vi "Main_old2.vi"() -> ()   [LabVIEW 2021]
uses:
  Enums/BatteryHealth_Enum.ctl
  Enums/Battery_Types.ctl
  Enums/States_Enum.ctl
  <vilib>/Utility/file.llb/Read Delimited Spreadsheet (DBL).vi
panel:
  out "counter":u8
  out "measurements done":u8
  out "Program State":T1
  in  "Battery Type":T2
  out "Quick Battery Health":T3
  out "error output":errorcluster
  in  "Stop Measurement":bool
  out "Battery Percentage":dbl caption="%" format="%#_2g%%"
  out "Internal Resistance":dbl format="%#_gohm"
  in  "Start Measurement":bool
  out "Battery Percentage Meter":dbl(knob)=21.586596923816817 caption="Meter" scale=0.0..100.0 scale format="%#_3g"
  out "read config":dbl[](array[numeric])
  out "read ascii file error":errorcluster
  in  "Terminate Run":bool
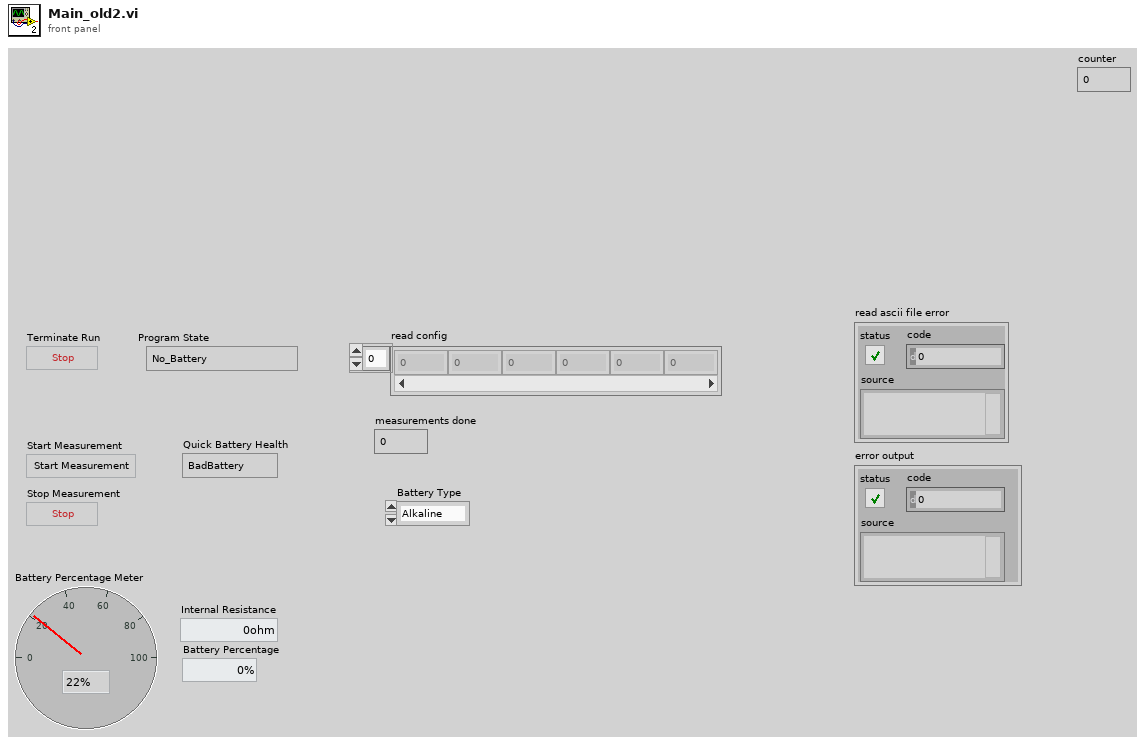
[diagram p1: front panel]
types:
  T1 = typedef "States_Enum.ctl" = enum16{"No_Battery", "Measure_loaded_circuit", "Stop_measurement", "Error"}
  T2 = typedef "Battery_Types.ctl" = enum16{"Alkaline", "Lithium"}
  T3 = typedef "BatteryHealth_Enum.ctl" = enum16{"BadBattery", "GoodBattery"}
  T4 = cluster{"no_load_voltage":dbl, "load_voltage":dbl, "load_voltage_percentage":dbl, "internal_resistance":dbl}
  T5 = typedef "Counter.ctl" = u8
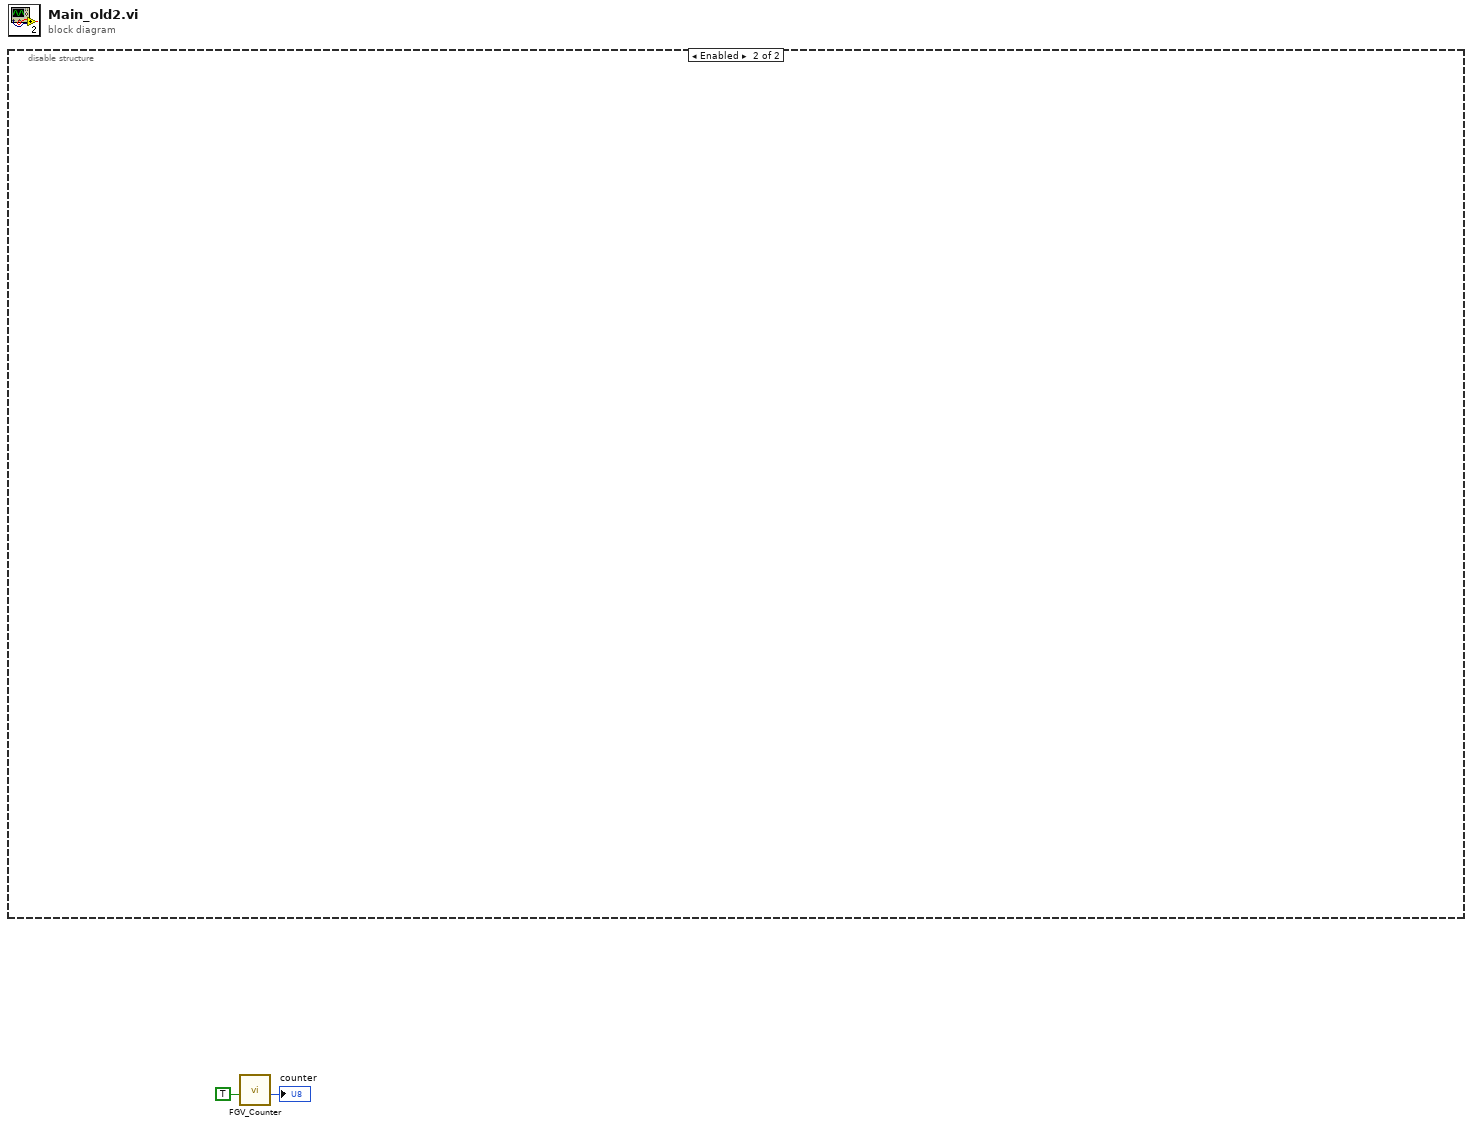
[diagram p0: block diagram]
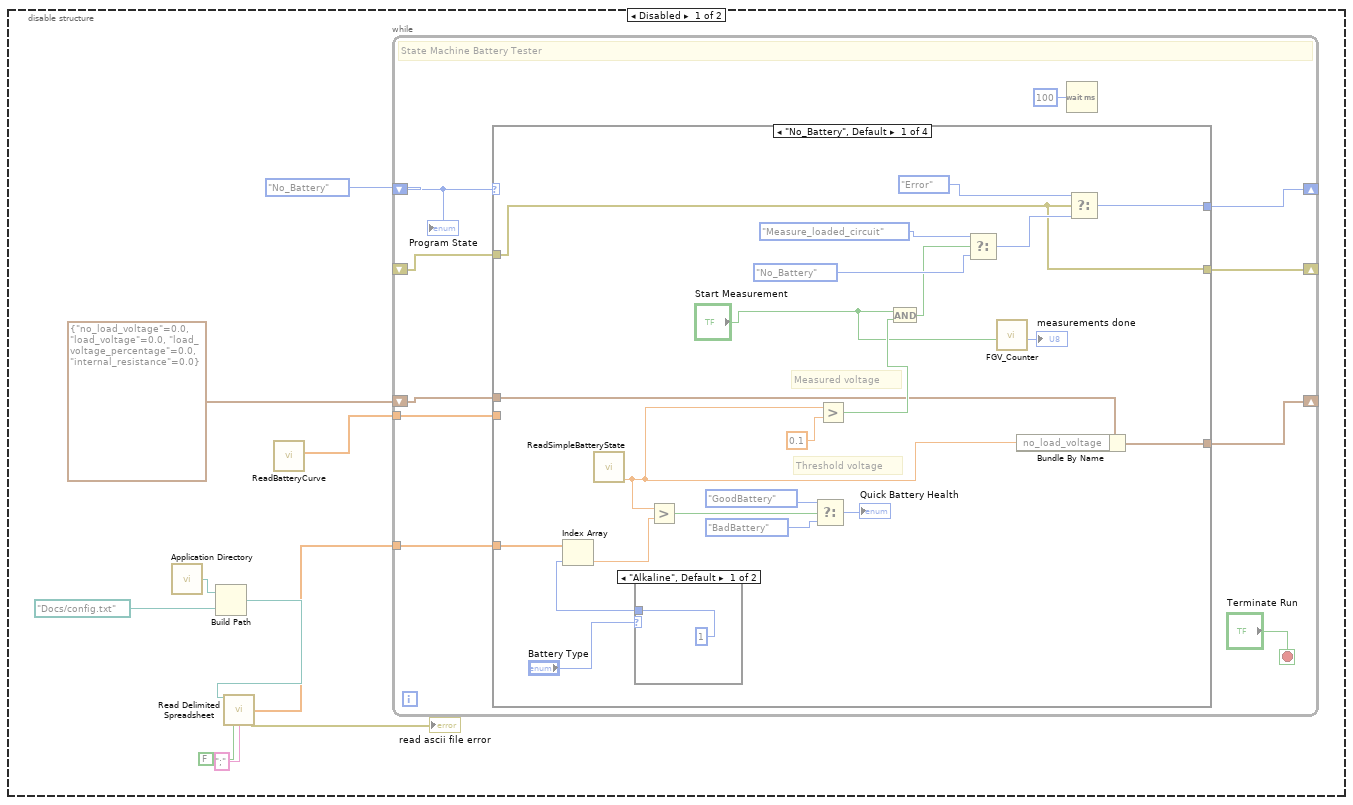
[diagram p2: hidden frame]
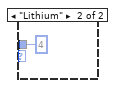
[diagram p3: hidden frame]
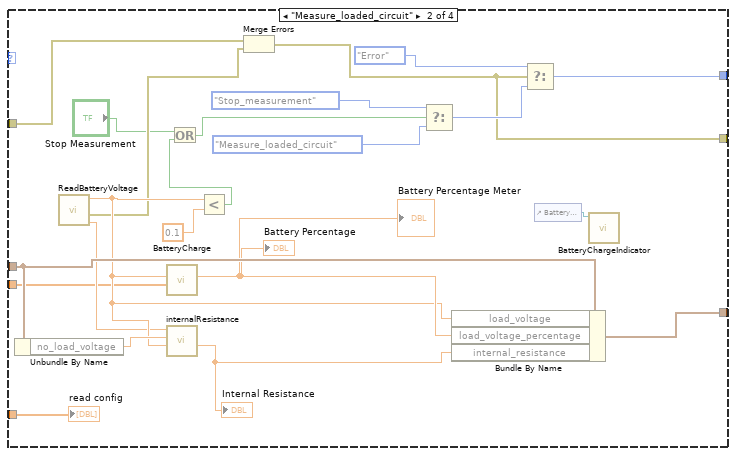
[diagram p4: hidden frame]
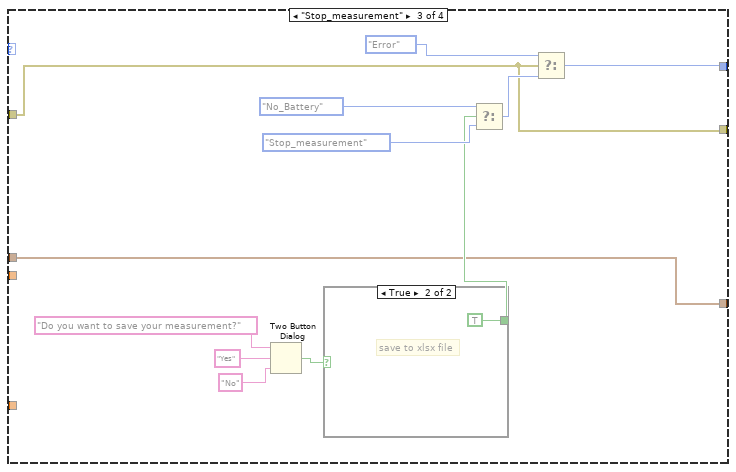
[diagram p5: hidden frame]
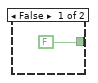
[diagram p6: hidden frame]
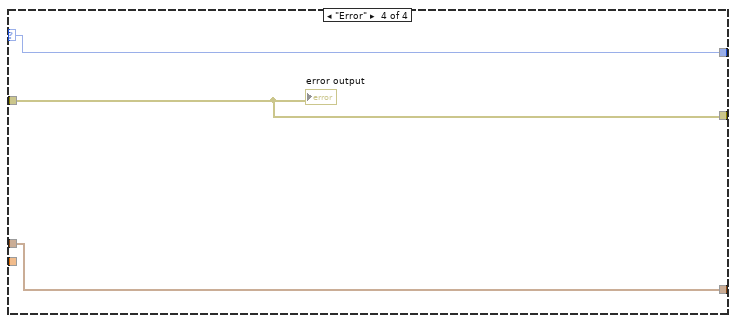
[diagram p7: hidden frame]
diagram:
  n1 = disable-structure shown="Enabled" {
    frame Disabled {
      n2 = call <vilib>:"Application Directory.vi"() -> ("Application Directory"=w8:path)
      n3 = Build Path(base path=w8, name or relative path=path "Docs/config.txt") -> (appended path=w6:path)
      n4 = call-poly <vilib>:"Read Delimited Spreadsheet.vi"("file path (dialog if empty)"=w6, "transpose? (F)"=FALSE, "delimiter (\\t)"=";" ("delimiter (\\t)")) -> ("first row"=w4:dbl[], "error out"=→"read ascii file error":errorcluster)  [unwired: 7 in, 4 out]
      n5 = call "ReadBatteryCurve.vi"() -> ("subarray 2"=w3:dbl[])  [unwired: 11 in]
      n6 = while "State Machine Battery Tester" {
        shift-right: [w19] -> _
        shift-left: States_Enum."No_Battery" ("Enum") -> [w20]
        shift-right: [w17] -> _
        shift-left: T4 {"no_load_voltage"=0.0, "load_voltage"=0.0, "load_voltage_percentage"=0.0, "internal_resistance"=0.0} -> [w18]
        shift-right: [w16] -> _
        shift-left: _ -> [w15]
        tunnel: w4 -> [w14]
        tunnel: w3 -> [w13]
        stop <- "Terminate Run" stop-if-true
        # "State Machine Battery Tester"
        n7 = case shown="\"No_Battery\", Default" w20 {
          selector: w20 -> [_ _ _ w85]
          tunnel: [w40 w65 w76 w85] -> w19
          tunnel: w18 -> [w33 w59 w69 w84]
          tunnel: [w36 w55 w69 w84] -> w17
          tunnel: [w35 w52 w70 w83] -> w16
          tunnel: w15 -> [w35 w54 w70 w83]
          tunnel: w14 -> [w32 w51 _ _]
          tunnel: w13 -> [_ w49 _ _]
          frame "No_Battery", Default {
            # "Threshold voltage"
            # "Measured voltage"
            n8 = call "ReadSimpleBatteryState.vi"() -> ("measurement"=w34:dbl)  [unwired: 11 in]
            n9 = case shown="\"Alkaline\", Default" "Battery Type" {
              tunnel: [1 ("index") 4 ("index")] -> w25
              frame "Alkaline", Default {
              }
              frame "Lithium" {
              }
            }
            n10 = Index Array(array=w32, index=w25) -> (element=w31:dbl)
            n11 = Greater?(x=w34, y=w31) -> (0:w30:bool)
            n12 = Select(t=BatteryHealth_Enum."GoodBattery" ("BatteryHealth"), s=w30, f=BatteryHealth_Enum."BadBattery" ("BatteryHealth")) -> (s? t:f=→"Quick Battery Health":T3)
            n13 = Greater?(x=w34, y=0.1) -> (0:w38:bool)
            n14 = And(x="Start Measurement", y=w38) -> (x .and. y?=w37:bool)
            n15 = Select(t=States_Enum."Measure_loaded_circuit" ("Enum"), s=w37, f=States_Enum."No_Battery" ("Enum")) -> (s? t:f=w44:T1)
            n16 = call "FGV_Counter.vi"("increment"="Start Measurement") -> ("counter"=→"measurements done":T5)  [unwired: 10 in]
            n17 = Bundle By Name(cluster=w33, "no_load_voltage"=w34) -> (w36:T4)
            n18 = Select(t=States_Enum."Error" ("Enum"), s=w35, f=w44) -> (s? t:f=w40:T1)
          }
          frame "Measure_loaded_circuit" {
            n19 = Unbundle By Name(w59) -> ("no_load_voltage"=w60:dbl)
            n20 = call "ReadBatteryVoltage.vi"() -> ("LoadCurrentFiltered"=w50:dbl, "error wirte/read"=w53:errorcluster, "BatteryVoltageFiltered"=w56:dbl)  [unwired: 8 in, 1 out]
            n21 = call "BatteryCharge.vi"("Battery_curve_array"=w49, "Measured_Voltage"=w56) -> ("Battery Percentage"=w58:dbl)  [unwired: 9 in]
            "Battery Percentage" <- w58
            "Battery Percentage Meter" <- w58
            n22 = call "internalResistance.vi"("loaded circuit voltage"=w56, "open circuit voltage"=w60, "Amperage over \nloaded curcuit"=w50) -> ("Internal resistance"=w57:dbl)  [unwired: 8 in]
            "Internal Resistance" <- w57
            n23 = Less?(x=w56, y=0.1) -> (x < y?=w63:bool)
            n24 = Or(x="Stop Measurement", y=w63) -> (x .or. y?=w62:bool)
            n25 = Merge Errors(w54, w53) -> (w52:errorcluster)
            n26 = Select(t=States_Enum."Stop_measurement" ("Enum"), s=w62, f=States_Enum."Measure_loaded_circuit" ("Enum")) -> (s? t:f=w61:T1)
            n27 = Bundle By Name(cluster=w59, "load_voltage"=w56, "load_voltage_percentage"=w58, "internal_resistance"=w57) -> (w55:T4)
            n28 = Select(t=States_Enum."Error" ("Enum"), s=w52, f=w61) -> (s? t:f=w65:T1)
            n29 = control-ref of="Battery Percentage Meter"() -> (w47:refnum<vi>)
            n30 = call "BatteryChargeIndicator.vi"("Knob in"=w47) -> ()  [unwired: 11 in]
            "read config" <- w51
          }
          frame "Stop_measurement" {
            n31 = Two Button Dialog(message="Do you want to save your measurement?", 1:"No" ("F button name (\"Cancel\")"), 2:"Yes" ("T button name (\"OK\")")) -> (T button?=w72:bool)
            n32 = case shown="True" w72 {
              tunnel: [FALSE TRUE] -> w71
              frame False {
              }
              frame True {
                # "save to xlsx file"
              }
            }
            n33 = Select(t=States_Enum."No_Battery" ("Enum"), s=w71, f=States_Enum."Stop_measurement" ("Enum")) -> (s? t:f=w80:T1)
            n34 = Select(t=States_Enum."Error" ("Enum"), s=w70, f=w80) -> (s? t:f=w76:T1)
          }
          frame "Error" {
            "error output" <- w83
          }
        }
        n35 = Wait (ms)(milliseconds to wait=u32 100) -> ()  [unwired: 1 out]
        "Program State" <- w20
      }
    }
    frame Enabled {
    }
  }
  n36 = call "FGV_Counter.vi"("increment"=TRUE) -> ("counter"=→"counter":T5)  [unwired: 10 in]
